vi "IDN.vi"(8 "Error In":errorcluster, 11 "VISA resource name":refnum<visa-resource-name>) -> (0 "Error Out":errorcluster, 2 "Read Data":string, 3 "VISA resource name out":refnum<visa-resource-name>)   [LabVIEW 2013]
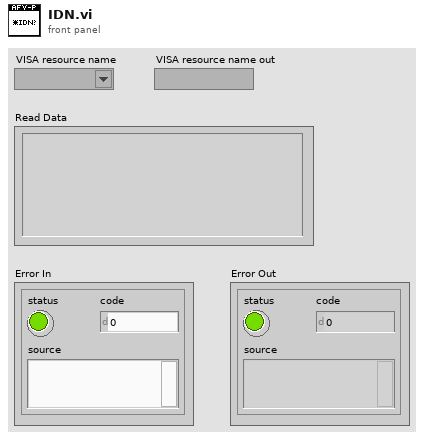
[diagram p1: front panel]
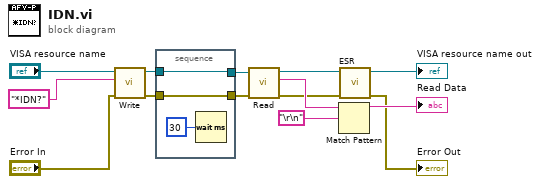
[diagram p0: block diagram]
diagram:
  n1 = call "Write.vi"("Error In"="Error In", "Write Buffer"="*IDN?", "VISA resource name"="VISA resource name") -> ("Error Out"=w9:errorcluster, "VISA resource name out"=w12:refnum<visa-resource-name>)  [unwired: 7 in]
  n2 = stacked-sequence {
    tunnel: [w16] -> w11
    tunnel: w12 -> [w16]
    tunnel: [w15] -> w10
    tunnel: w9 -> [w15]
    frame #0 {
      n3 = Wait (ms)(milliseconds to wait=u32 30) -> ()  [unwired: 1 out]
    }
  }
  n4 = call "Read.vi"("Error In"=w10, "VISA resource name"=w11) -> ("Error Out"=w4:errorcluster, "Read Data"=w5:string, "VISA resource name out"=w2:refnum<visa-resource-name>)  [unwired: 7 in]
  n5 = Match Pattern(string=w5, regular expression="\r\n") -> (before substring=→"Read Data":string)  [unwired: 1 in, 3 out]
  n6 = call "ESR.vi"("Error In"=w4, "VISA resource name"=w2) -> ("Error Out"=→"Error Out":errorcluster, "VISA resource name out"=→"VISA resource name out":refnum<visa-resource-name>)  [unwired: 8 in]
